vi "Create User Events FGV.vi"(8 "error in":errorcluster, 11 "Initialize":bool) -> (0 "error out":errorcluster, 3 "User Events":T1)   [LabVIEW 2019, in "User Events.lvlib"]
doc: "Create a boolean user event that will be used to stop the event loop from the message handling loop."
uses:
  User Events.lvlib
  User Events Typedef.ctl
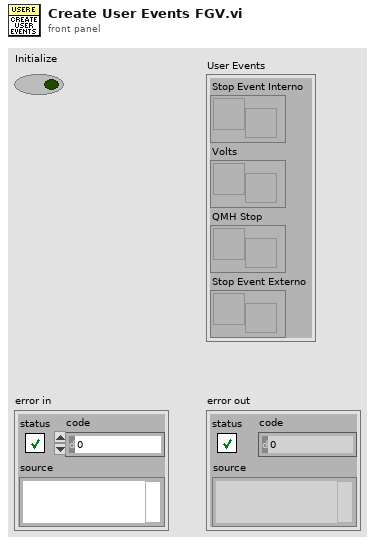
[diagram p1: front panel]
types:
  T1 = typedef "User Events.lvlib/User Events Typedef.ctl" = cluster{"Stop Event Interno":refnum<user-event>, "Volts":refnum<user-event>, "QMH Stop":refnum<user-event>, "Stop Event Externo":refnum<user-event>}
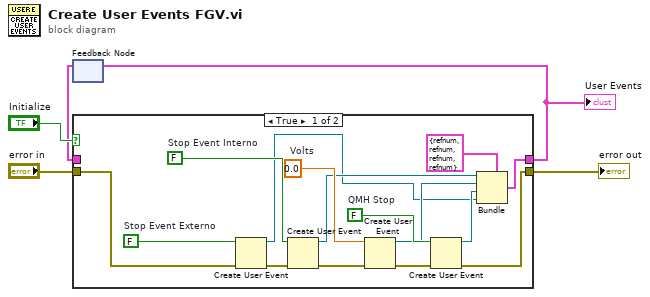
[diagram p0: block diagram]
diagram:
  n1 = feedback #1() -> (w1:T1)  [unwired: 1 in]
  n2 = case shown="True" "Initialize" {
    tunnel: [w11 w21] -> w2
    tunnel: [w18 w22] -> w5
    tunnel: "error in" -> [w8 w22]
    tunnel: w1 -> [_ w21]
    frame True {
      w9 = FALSE  # Stop Event Externo
      w15 = FALSE  # QMH Stop
      w16 = 0.0  # Volts
      w17 = FALSE  # Stop Event Interno
      n3 = Create User Event(user event datatype=w9, error in=w8) -> (user event=w6:refnum<user-event>, error out=w7:errorcluster)
      n4 = Create User Event(user event datatype=w17, error in=w7) -> (user event=w14:refnum<user-event>, error out=w20:errorcluster)
      n5 = Create User Event(user event datatype=w16, error in=w20) -> (user event=w13:refnum<user-event>, error out=w19:errorcluster)
      n6 = Create User Event(user event datatype=w15, error in=w19) -> (user event=w12:refnum<user-event>, error out=w18:errorcluster)
      n7 = Bundle(cluster=T1 {"Stop Event Interno"=refnum, "Volts"=refnum, "QMH Stop"=refnum, "Stop Event Externo"=refnum} ("User Events"), "Stop Event Interno"=w14, "Volts"=w13, "QMH Stop"=w12, "Stop Event Externo"=w6) -> (w11:T1)
    }
    frame False {
    }
  }
  "error out" <- w5
  "User Events" <- w2
  n8 = feedback-in #1(w2) -> ()
